vi "Draw Image.vi"() -> ()   [LabVIEW 2020]
panel:
  in  "Color Box":u32(colorbox)
  in  "Array":u32[][](array[colorbox])
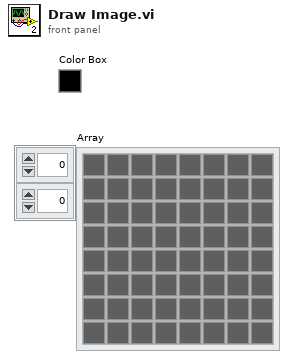
[diagram p1: front panel]
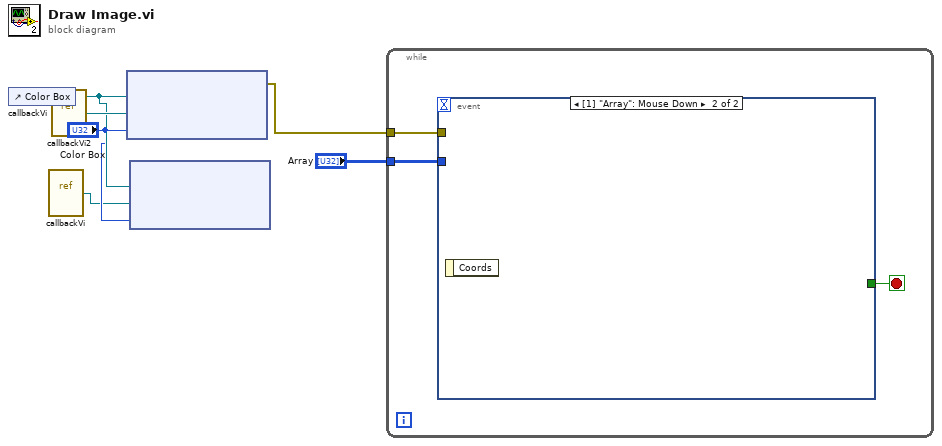
[diagram p0: block diagram]
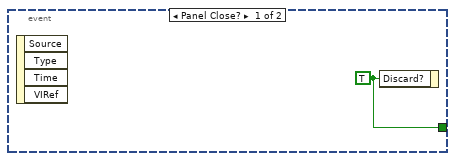
[diagram p2: hidden frame]
diagram:
  n1 = control-ref of="Color Box"() -> (w3:refnum<vi>)
  n2 = vi-ref "callbackVi.vi"() -> ("vi reference"=w1:refnum<vi>)
  n3 = vi-ref "callbackVi2.vi"() -> ("vi reference"=w4:refnum<vi>)
  n4 = vi-ref "callbackVi.vi"() -> ()  [unwired: 1 out]
  n5 = node(w3, w4, "Color Box") -> (w5:errorcluster)  [unwired: 2 in, 1 out]
  n6 = node(w3, w1, "Color Box") -> ()  [unwired: 2 in, 2 out]
  n7 = while {
    tunnel: "Array" -> [w9]
    tunnel: w5 -> [w7]
    stop <- w8 stop-if-true
    n8 = event shown="[1] \"Array\": Mouse Down" {
      selector: _ -> [_ _]
      dyn-events: _ -> [_ _]
      timeout: _ -> [_ _]
      tunnel: w9 -> [_ _]
      tunnel: [w10 _] -> w8
      tunnel: w7 -> [_ _]
      event Panel Close? {
        w10 = TRUE ("Discard?")
        n9 = event-data() -> ()  [unwired: 1 in, 4 out]
        n10 = event-data("Discard?"=w10) -> ()  [unwired: 1 in, 1 out]
      }
      event "Array": Mouse Down {
        n11 = event-data() -> ()  [unwired: 1 in, 1 out]
      }
    }
  }
